vi "Untitled 18.vi"() -> ()   [LabVIEW 2015]
uses:
  Type Definitions/control_references.ctl
  Type Definitions/vars_settings.ctl
panel:
  in  "error in (no error)":errorcluster
  out "error out":errorcluster
  in  "vars general in":T1[](array[typedef])
  in  "control cluster in":T2
  out "vars general out":T1[](array[typedef])
  out "control cluster out":T2
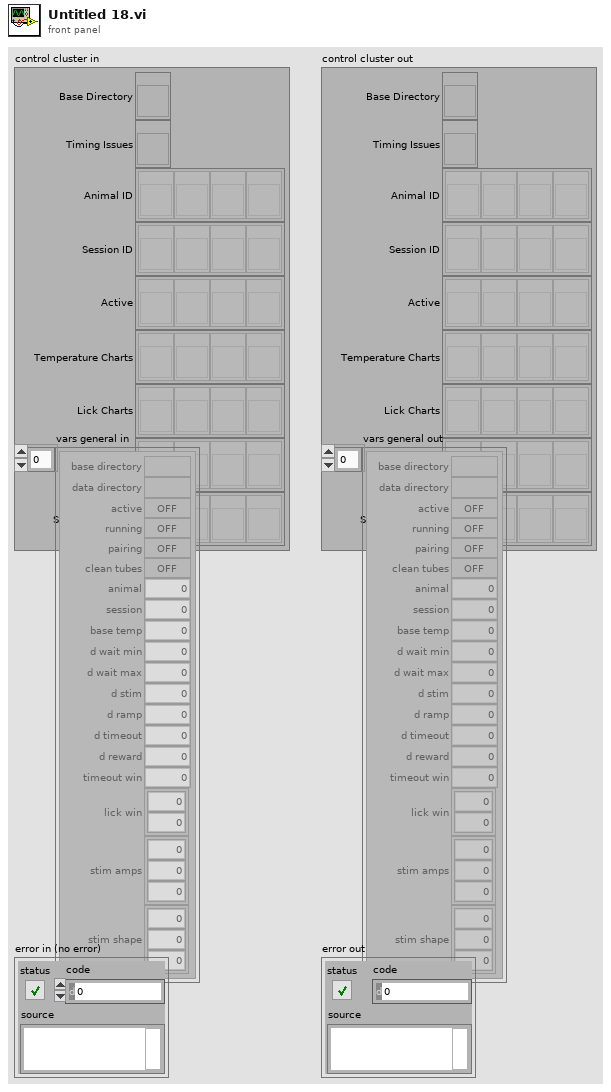
[diagram p1: front panel]
types:
  T1 = typedef "vars_settings.ctl" = cluster{"base directory":path, "data directory":path, "active":bool, "running":bool, "pairing":bool, "clean tubes":bool, "animal":u16, "session":u16, "base temp":sgl, "d wait min":u16, "d wait max":u16, "d stim":u16, "d ramp":u16, "d timeout":u16, "d reward":u16, "timeout win":u16, "lick win":i32[], "stim amps":dbl[], "stim shape":dbl[]}
  T2 = typedef "control_references.ctl" = cluster{"Base Directory":refnum<vi>, "Timing Issues":refnum<vi>, "Animal ID":refnum<vi>[], "Session ID":refnum<vi>[], "Active":refnum<vi>[], "Temperature Charts":refnum<vi>[], "Lick Charts":refnum<vi>[], "Bool Displays":refnum<vi>[], "Stimulus Timing":refnum<vi>[]}
  T3 = enum8{"Enabled", "Disabled", "Disabled and Grayed Out"}
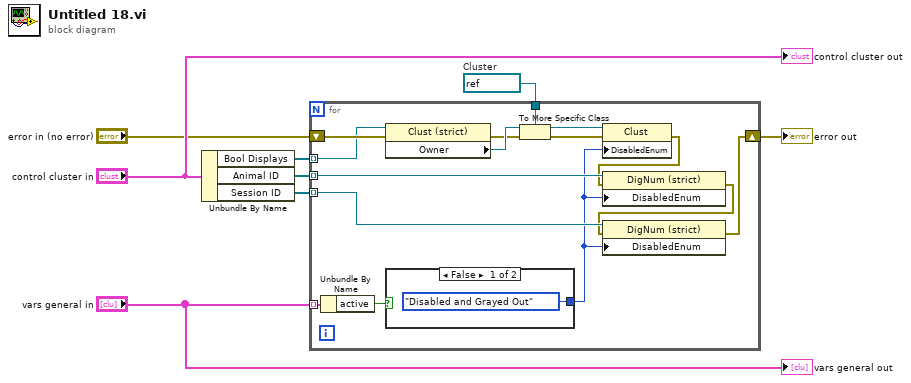
[diagram p0: block diagram]
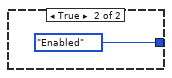
[diagram p2: hidden frame]
diagram:
  w7 = refnum<vi> refnum  # Cluster
  n1 = Unbundle By Name("control cluster in") -> ("Bool Displays"=w3:refnum<vi>[], "Animal ID"=w2:refnum<vi>[], "Session ID"=w1:refnum<vi>[])
  n2 = for {
    tunnel: w7 -> [w19]
    shift-right: [w9] -> w5
    shift-left: "error in (no error)" -> [w18]
    tunnel: "vars general in" -> [w16] mode=indexing
    tunnel: w3 -> [w15] mode=indexing
    tunnel: w2 -> [w14] mode=indexing
    tunnel: w1 -> [w13] mode=indexing
    n3 = Unbundle By Name(w16) -> ("active"=w17:bool)
    n4 = property class="Clust (strict)"(reference=w15, error in=w18) -> (error out=w20:errorcluster, "Owner"=w23:refnum<vi>)  [unwired: 1 out]
    n5 = case shown="False" w17 {
      tunnel: [T3."Disabled and Grayed Out" ("Disabled") T3."Enabled" ("Disabled")] -> w12
      frame False {
      }
      frame True {
      }
    }
    n6 = To More Specific Class(target class=w19, reference=w23, error in=w20) -> (specific class reference=w22:refnum<vi>, error out=w21:errorcluster)
    n7 = property class="Clust"(reference=w22, error in=w21, "DisabledEnum"=w12) -> (error out=w11:errorcluster)  [unwired: 1 out]
    n8 = property class="DigNum (strict)"(reference=w14, error in=w11, "DisabledEnum"=w12) -> (error out=w10:errorcluster)  [unwired: 1 out]
    n9 = property class="DigNum (strict)"(reference=w13, error in=w10, "DisabledEnum"=w12) -> (error out=w9:errorcluster)  [unwired: 1 out]
  }
  "error out" <- w5
  "control cluster out" <- "control cluster in"
  "vars general out" <- "vars general in"
